vi "PCI1220U扭矩轴读取位置.vi"(11 "AxisHandle IN":u32) -> (2 "位置":dbl=10000.0, 3 "AxisHandle OUT":u32)   [LabVIEW 2013]
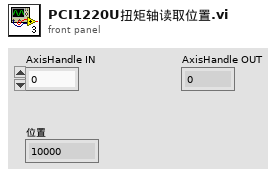
[diagram p1: front panel]
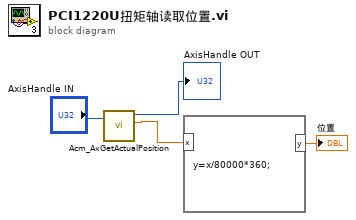
[diagram p0: block diagram]
diagram:
  n1 = call <userlib>:"Acm_AxGetActualPosition.vi"("AxisHandle"="AxisHandle IN") -> ("Position"=w1:dbl, "AxisHandle"=→"AxisHandle OUT":u32)  [unwired: 1 in, 2 out]
  n2 = formula code="y=x/80000*360;"("x"=w1) -> ("y"=→"位置":dbl)
